vi "XY to Rotated Pixel Points.vi"(4 "use roll":bool=TRUE, 6 "use pitch":bool=TRUE, 7 "attitude (rad)":T1, 9 "draw area state":T2, 10 "unrotated y (units)":dbl[](array[numeric]), 11 "unrotated x (units)":dbl[](array[numeric])) -> (3 "rotated pixel points":cluster{"x":i16, "y":i16}[](array[cluster]))   [LabVIEW 2017, in "NI_Robotics_Attitude Picture.lvlib"]
uses:
  <vilib>/robotics/Controls/Attitude Indicator/Attitude Picture/NI_Robotics_Attitude Picture.lvlib
  <vilib>/robotics/Controls/Attitude Indicator/Attitude Picture/Draw Area State.ctl
  <vilib>/Utility/miscctls.llb/LVBoundsTypeDef.ctl
  <vilib>/robotics/Controls/Attitude Indicator/Attitude Picture/Attitude.ctl
  <vilib>/Analysis/coordinate.llb/2D Cartesian Coordinate Rotation (Array).vi
  <vilib>/Analysis/NI_AALPro.lvlib
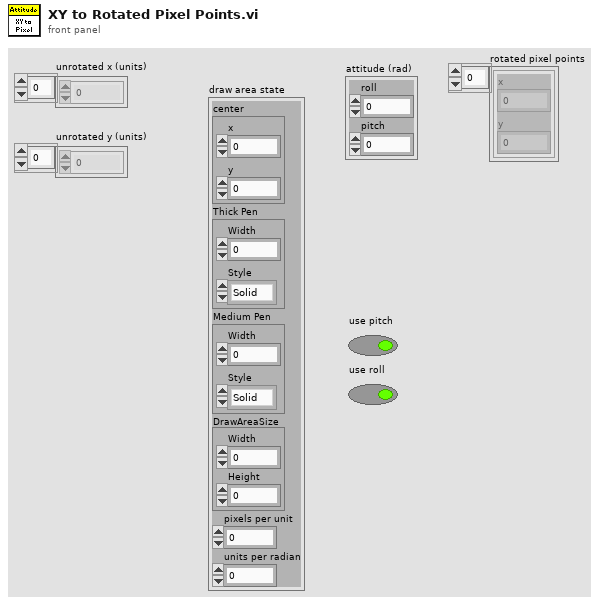
[diagram p1: front panel]
types:
  T1 = typedef "NI_Robotics_Attitude Picture.lvlib/Attitude.ctl" = cluster{"roll":dbl, "pitch":dbl}
  T2 = typedef "NI_Robotics_Attitude Picture.lvlib/Draw Area State.ctl" = cluster{"center":cluster{"x":i16, "y":i16}, "Thick Pen":cluster{"Width":u16, "Style":enum32{"Solid", "Dash", "Dot", "DashDot", "DashDotDot"}}, "Medium Pen":cluster{"Width":u16, "Style":enum32{"Solid", "Dash", "Dot", "DashDot", "DashDotDot"}}, "DrawAreaSize":T3, "pixels per unit":dbl, "units per radian":dbl}
  T3 = typedef "LVBoundsTypeDef.ctl" = cluster{"Width":u32, "Height":u32}
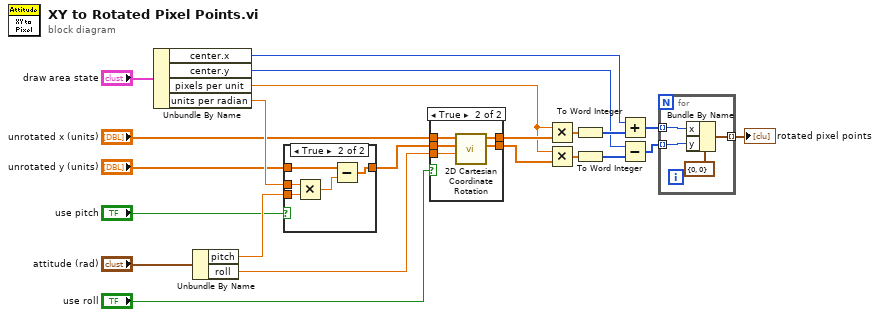
[diagram p0: block diagram]
diagram:
  n1 = Unbundle By Name("draw area state") -> ("center.x"=w4:i16, "center.y"=w5:i16, "pixels per unit"=w6:dbl, "units per radian"=w19:dbl)
  n2 = Unbundle By Name("attitude (rad)") -> ("pitch"=w20:dbl, "roll"=w15:dbl)
  n3 = case shown="True" "use pitch" {
    tunnel: w20 -> [_ w28]
    tunnel: w19 -> [_ w27]
    tunnel: "unrotated y (units)" -> [w23 w26]
    tunnel: [w23 w24] -> w16
    frame False {
    }
    frame True {
      n4 = Multiply(x=w27, y=w28) -> (x*y=w25:dbl)
      n5 = Subtract(x=w26, y=w25) -> (x-y=w24:dbl[])
    }
  }
  n6 = case shown="True" "use roll" {
    tunnel: "unrotated x (units)" -> [w30 w35]
    tunnel: w16 -> [w29 w34]
    tunnel: w15 -> [_ w33]
    tunnel: [w30 w32] -> w8
    tunnel: [w29 w31] -> w7
    frame False {
    }
    frame True {
      n7 = call-poly <vilib>:"2D Cartesian Coordinate Rotation.vi"("theta"=w33, "Y"=w34, "X"=w35) -> ("Y Out"=w31:dbl[], "X Out"=w32:dbl[])  [unwired: 6 in, 1 out]
    }
  }
  n8 = Multiply(x=w6, y=w8) -> (x*y=w10:dbl[])
  n9 = Multiply(x=w6, y=w7) -> (x*y=w9:dbl[])
  n10 = To Word Integer(number=w10) -> (16bit integer=w13:i16[])
  n11 = To Word Integer(number=w9) -> (16bit integer=w14:i16[])
  n12 = Add(x=w4, y=w13) -> (x+y=w12:i16[])
  n13 = Subtract(x=w5, y=w14) -> (x-y=w11:i16[])
  n14 = for {
    tunnel: w12 -> [w38] mode=indexing
    tunnel: w11 -> [w37] mode=indexing
    tunnel: [w36] -> w3 mode=indexing
    n15 = Bundle By Name(cluster=cluster{"x":i16, "y":i16} {"x"=0, "y"=0}, "x"=w38, "y"=w37) -> (w36:cluster{"x":i16, "y":i16})
  }
  "rotated pixel points" <- w3
